vi "Stop VIs Stream.vi"(8 "error in (no error)":errorcluster, 11 "Channel in":refnum<class "Channel.lvclass">) -> (0 "error out":errorcluster, 3 "Channel out":refnum<class "Channel.lvclass">)   [LabVIEW 2018, in "Channel.lvclass"]
uses:
  Channel.lvclass
  Channel.lvclass/Channel.ctl
  RxTx/RxTx.lvclass
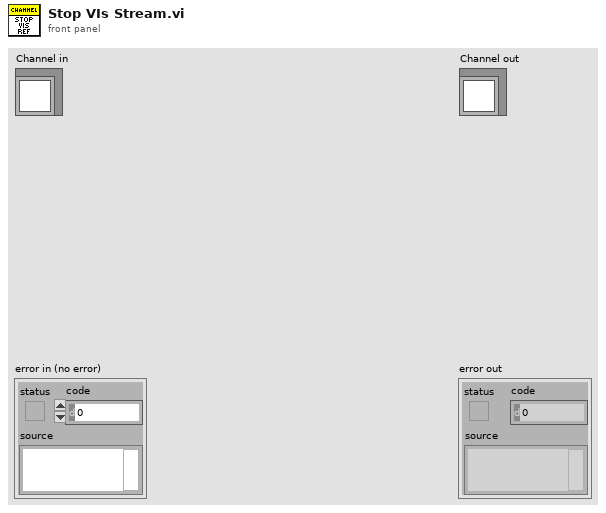
[diagram p1: front panel]
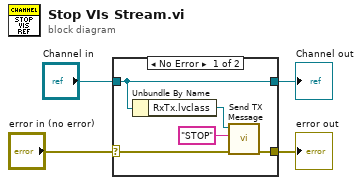
[diagram p0: block diagram]
diagram:
  n1 = case shown="No Error" "error in (no error)" {
    selector: "error in (no error)" -> [w6 w11]
    tunnel: [w7 w11] -> w3
    tunnel: [w9 w10] -> w1
    tunnel: "Channel in" -> [w9 w10]
    frame No Error {
      n2 = Unbundle By Name(w9) -> ("RxTx.lvclass"=w8:refnum<class "RxTx.lvclass">)
      n3 = call "Send TX Message.vi"("error in (no error)"=w6, "element"="STOP", "RxTx in"=w8) -> ("error out"=w7:errorcluster)  [unwired: 7 in, 1 out]
    }
    frame Error {
    }
  }
  "error out" <- w3
  "Channel out" <- w1
